vi "UI.vi"() -> ()   [LabVIEW 2014]
uses:
  <vilib>/rvi/interface/nirviOpenFPGA/nirviOpenFPGA.xnode
  FPGA Target/Top Level FPGA.vi
panel:
  out "ERROR":bool
  in  "Wave values path":path
  out "Speed":dbl
  out "Distance":dbl
  in  "Running":bool
  in  "Start/Stop":bool
  # "Configuration"
  # "Run"
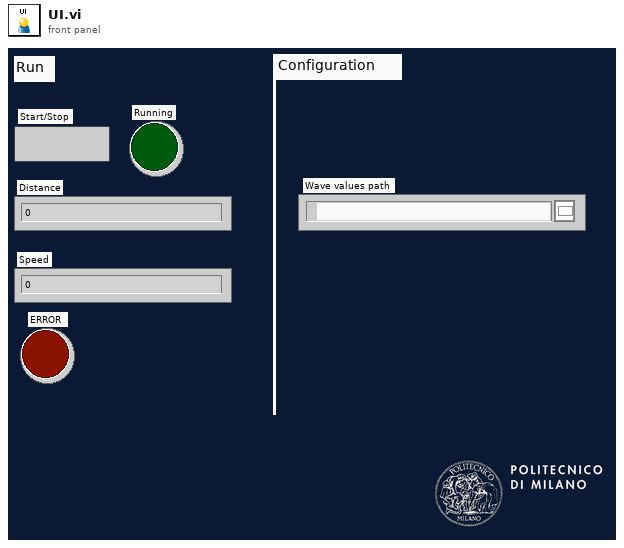
[diagram p1: front panel]
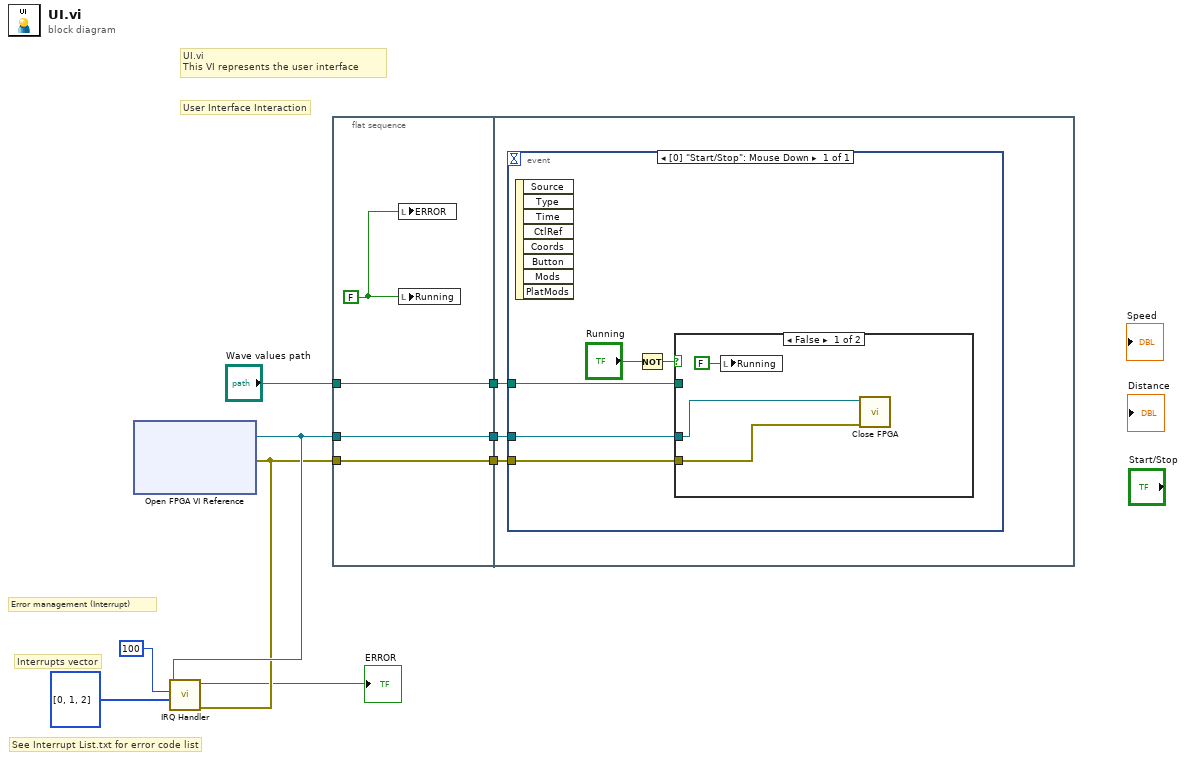
[diagram p0: block diagram]
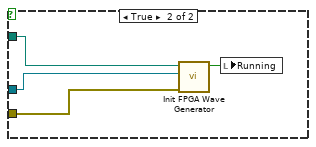
[diagram p2: hidden frame]
diagram:
  # "See Interrupt List.txt for error code list"
  # "Interrupts vector"
  # "Error management (Interrupt)"
  # "UI.vi\nThis VI represents the user interface"
  # "User Interface Interaction"
  n1 = xnode "Open FPGA VI Reference"() -> ("FPGA VI Reference Out"=w5:refnum<k20>, "error out"=w4:errorcluster)  [unwired: 2 in]
  n2 = call "IRQ Handler.vi"("error in"=w4, "IRQ(s) Asserted"=i32[] [0, 1, 2], "Timeout (ms)"=100, "FPGA VI Reference In"=w5) -> ("IRQ occurred"=→"ERROR":bool)  [unwired: 7 in]
  n3 = flat-sequence {
    tunnel: [w13] -> w9
    tunnel: "Wave values path" -> [w13]
    tunnel: [w12] -> w7
    tunnel: w5 -> [w12]
    tunnel: [w11] -> w6
    tunnel: w4 -> [w11]
    tunnel: w9 -> [w16]
    tunnel: w7 -> [w15]
    tunnel: w6 -> [w14]
    frame #0 {
      w10 = FALSE ("Running")
      n4 = local write "ERROR"(w10) -> ()
      n5 = local write "Running"(w10) -> ()
    }
    frame #1 {
      n6 = event shown="[0] \"Start/Stop\": Mouse Down" {
        selector: _ -> [_]
        dyn-events: _ -> [_]
        timeout: _ -> [_]
        tunnel: w16 -> [w19]
        tunnel: w15 -> [w18]
        tunnel: w14 -> [w17]
        event "Start/Stop": Mouse Down {
          n7 = event-data() -> ()  [unwired: 1 in, 8 out]
          n8 = Not(x="Running") -> (.not. x?=w20:bool)
          n9 = case shown="False" w20 {
            tunnel: w19 -> [_ w27]
            tunnel: w18 -> [w22 w25]
            tunnel: w17 -> [w23 w26]
            frame False {
              n10 = local write "Running"(FALSE ("Running")) -> ()
              n11 = call "Close FPGA.vi"("error in"=w23, "FPGA VI Reference In"=w22) -> ()  [unwired: 9 in, 1 out]
            }
            frame True {
              n12 = call "Init FPGA Wave Generator.vi"("error in"=w26, "FPGA VI Reference In"=w25, "Wave path"=w27) -> ("Done"=w28:bool)  [unwired: 8 in]
              n13 = local write "Running"(w28) -> ()
            }
          }
        }
      }
    }
  }
